vi "Evaluate Concentration.vi"(5 "python in":refnum<k35>, 6 "List Concentration In":T1(array[cluster]) {"N. Peak" items=["0.000000", "1.000000", "2.000000", "3.000000", "4.000000", "5.000000", "6.000000", "7.000000", "8.000000", "9.000000", "10.000000", "11.000000", "12.000000", "13.000000", "14.000000", "15.000000", "16.000000", "17.000000", "18.000000", "19.000000", "20.000000", "21.000000", "22.000000", "23.000000", "24.000000", "25.000000", "26.000000", "27.000000", "28.000000"]}, 7 "Type Conentration":enum32{"Item 0", "Item 1"}(radio), 8 "error in":errorcluster, 9 "List ROI in":dbl[][](array[numeric]), 10 "Parameters In":T3[](array[typedef]), 11 "Elements Selected":string[][](table)) -> (0 "error out":errorcluster, 3 "Concentration":T2, 4 "python out":refnum<k35>)   [LabVIEW 2023]
uses:
  control/Parameters.ctl
  control/Concentrations.ctl
  e2a7fa98-077b-4280-a056-373c7a60fd3a.vi
  1848effe-5ca7-4314-be89-901603a86480.vi
  8bf43f8d-2068-40c8-874a-5f9a9f6e8e88.vi
  <vilib>/Comparison/Equal/Equal Functor/Equal Functor.lvclass
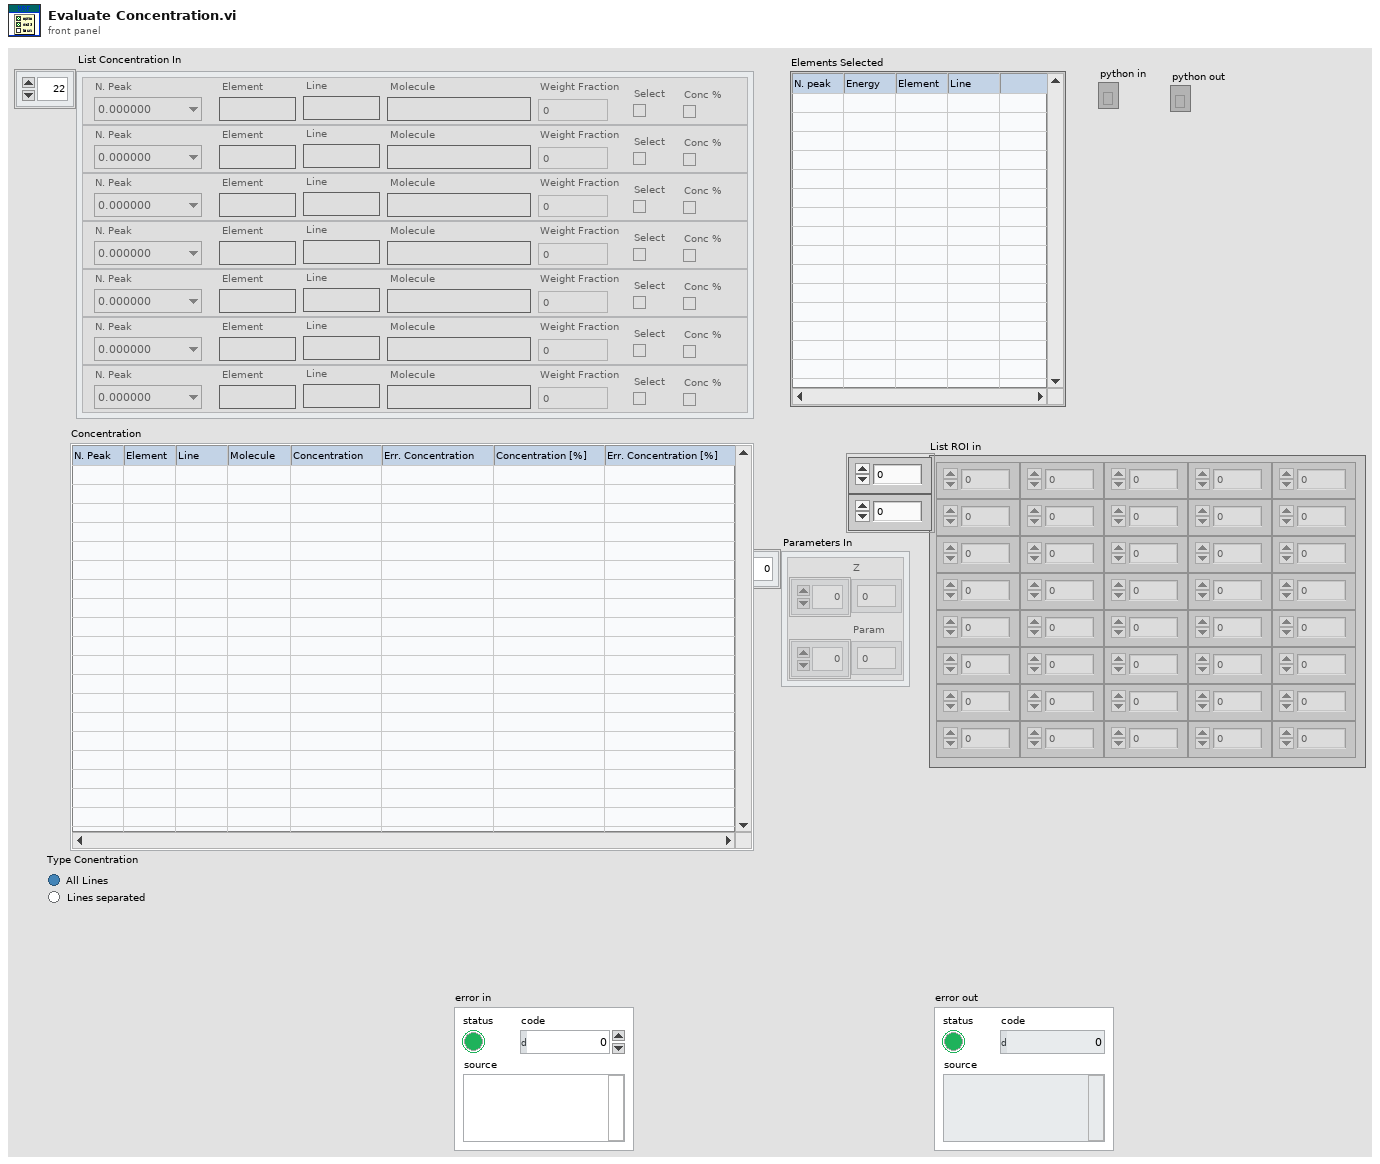
[diagram p1: front panel]
types:
  T1 = cluster{"N. Peak":u16, "Element":string, "Molecule":string, "Weight Fraction":dbl, "Select":bool, "Conc %":bool, "Line":string}[]
  T2 = typedef "Concentrations.ctl" = string[][]
  T3 = typedef "Parameters.ctl" = cluster{"Z":i32[], "Param":dbl[]}
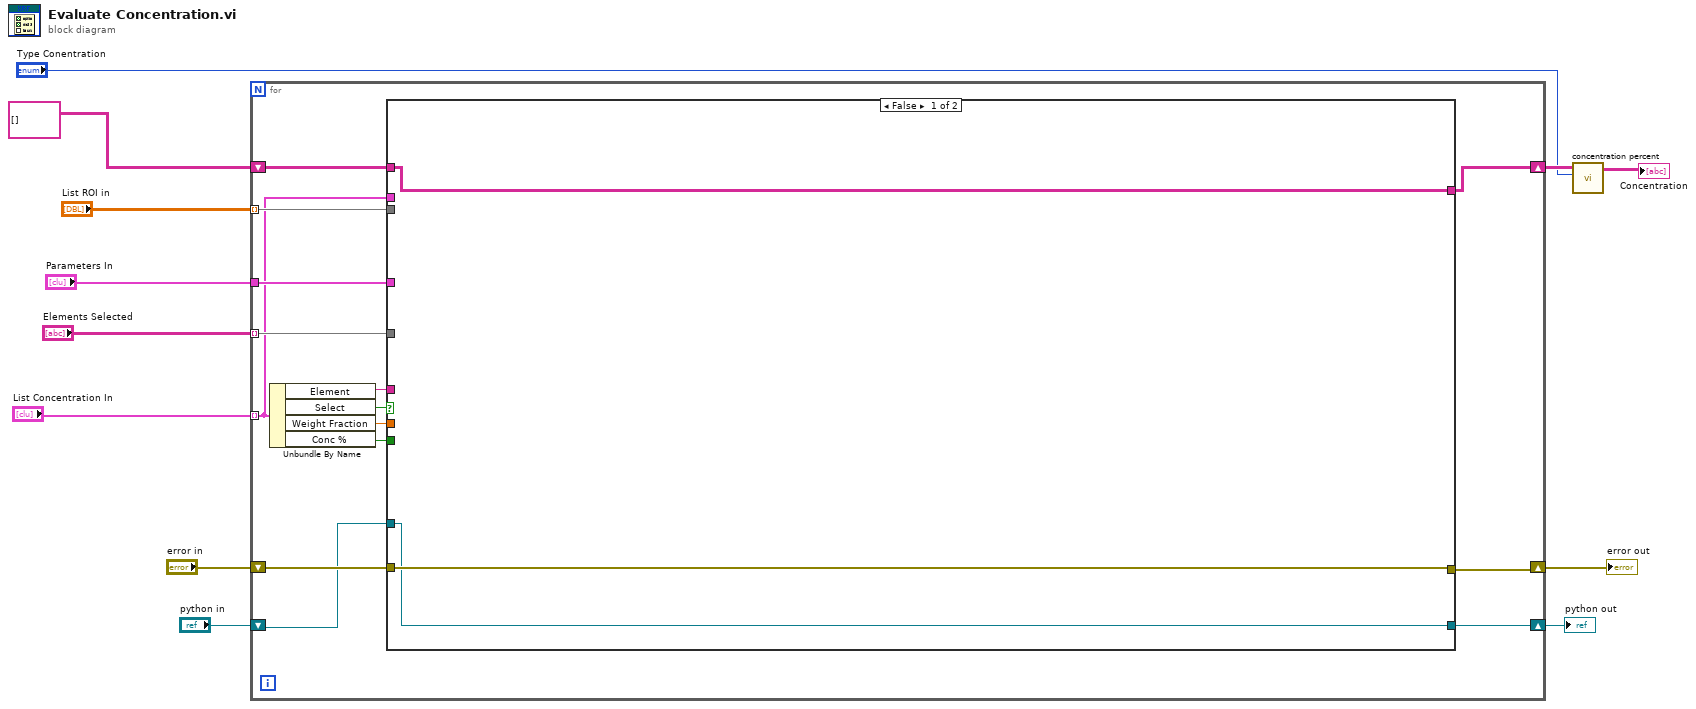
[diagram p0: block diagram]
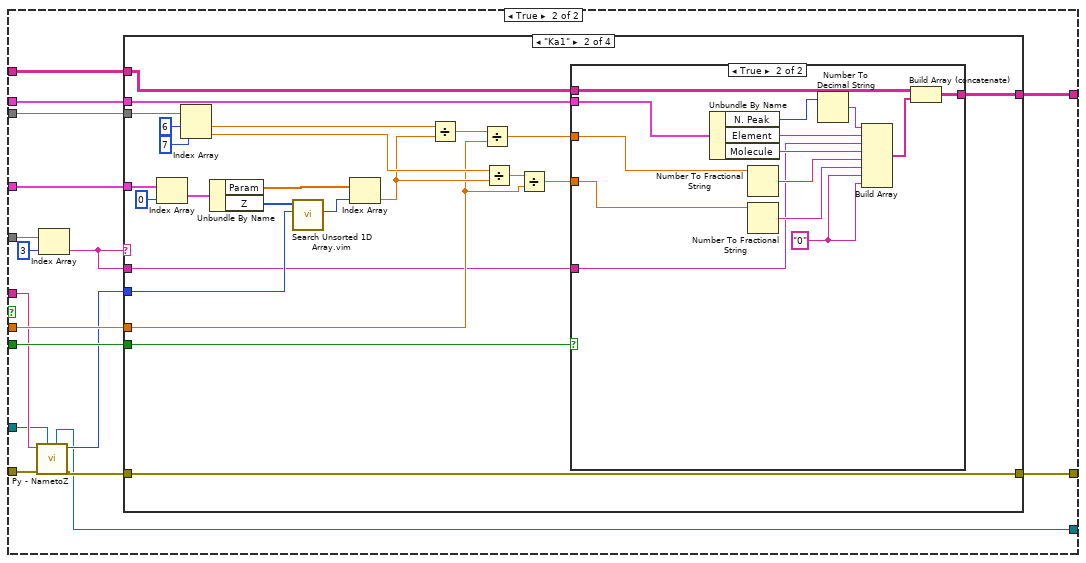
[diagram p2: hidden frame]
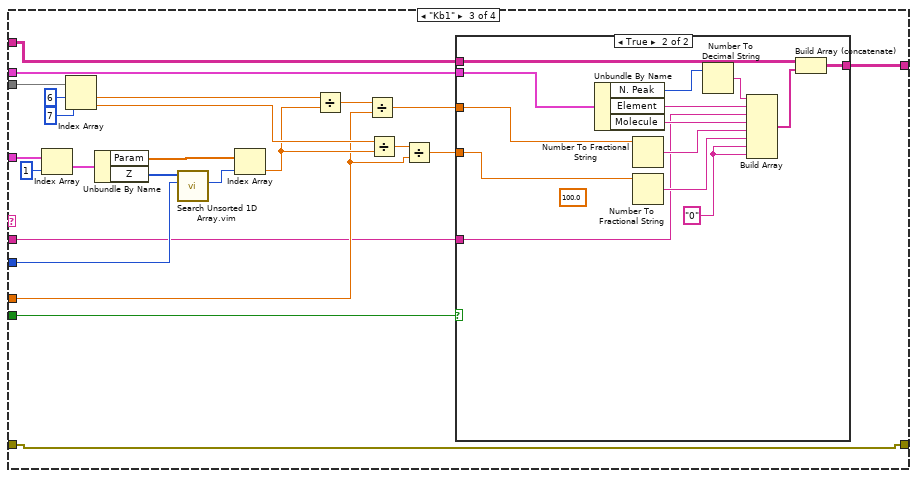
[diagram p5: hidden frame]
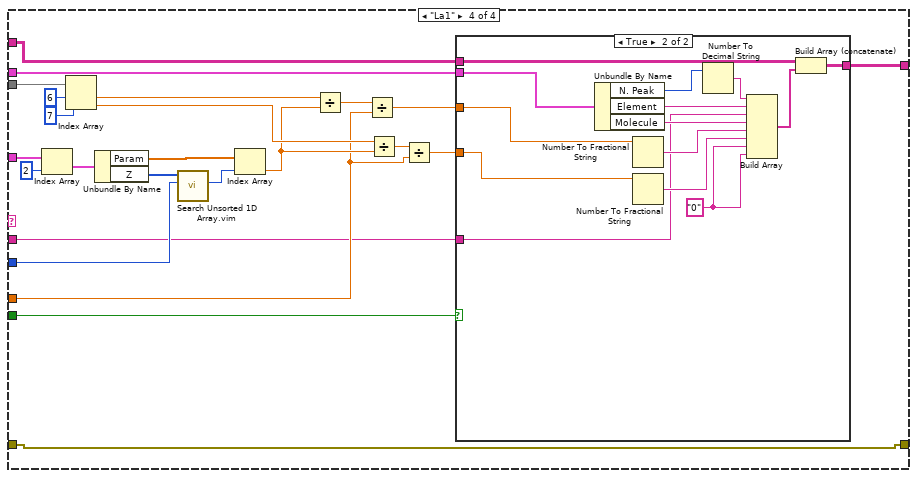
[diagram p7: hidden frame]
diagram:
  n1 = for {
    tunnel: "List Concentration In" -> [w18] mode=indexing
    tunnel: "Elements Selected" -> [w25] mode=indexing
    tunnel: "Parameters In" -> [w24]
    tunnel: "List ROI in" -> [w22] mode=indexing
    shift-right: [w17] -> w8
    shift-left: T2 [] ("Concentration") -> [w19]
    shift-right: [w15] -> w3
    shift-left: "error in" -> [w16]
    shift-right: [w14] -> w2
    shift-left: "python in" -> [w13]
    n2 = Unbundle By Name(w18) -> ("Element"=w23:string, "Select"=w26:bool, "Weight Fraction"=w21:dbl, "Conc %"=w20:bool)
    n3 = case shown="False" w26 {
      tunnel: w25 -> [_ w46]
      tunnel: w24 -> [_ w44]
      tunnel: w23 -> [_ w33]
      tunnel: w22 -> [_ w43]
      tunnel: w21 -> [_ w42]
      tunnel: w20 -> [_ w41]
      tunnel: w19 -> [w29 w40]
      tunnel: w18 -> [_ w39]
      tunnel: [w29 w38] -> w17
      tunnel: w16 -> [w28 w35]
      tunnel: [w28 w36] -> w15
      tunnel: [w27 w31] -> w14
      tunnel: w13 -> [w27 w30]
      frame False {
      }
      frame True {
        n4 = call "Py - NametoZ.vi"("python in"=w30, "error in"=w35, "Name Element"=w33) -> ("error out"=w34:errorcluster, "Z"=w32:i32, "python out"=w31:refnum<k35>)  [unwired: 6 in]
        n5 = Index Array(array=w46, index=3) -> (element=w37:string)
        n6 = case shown="\"Ka1\"" w37 {
          tunnel: w44 -> [_ w72 w111 w150]
          tunnel: w32 -> [_ w69 w108 w147]
          tunnel: w43 -> [_ w65 w104 w143]
          tunnel: w42 -> [_ w57 w96 w135]
          tunnel: w41 -> [_ w56 w95 w134]
          tunnel: w40 -> [w48 w54 w93 w132]
          tunnel: w39 -> [_ w55 w94 w133]
          tunnel: [w48 w51 w90 w129] -> w38
          tunnel: w37 -> [_ w50 w89 w128]
          tunnel: [w47 w49 w88 w127] -> w36
          tunnel: w34 -> [w47 w49 w88 w127]
          frame Default {
          }
          frame "Ka1" {
            n7 = Index Array(array=w72, index=0) -> (element=w70:T3)
            n8 = Index Array(array=w65, index #1=6 ("index"), index #2=7 ("index")) -> (element #1=w62:dbl, element #2=w59:dbl)
            n9 = Unbundle By Name(w70) -> ("Param"=w67:dbl[], "Z"=w68:i32[])
            n10 = call "Search Unsorted 1D Array.vim"("element"=w69, "unsorted 1D array"=w68) -> ("index of element"=w66:i32)  [unwired: 9 in]
            n11 = Index Array(array=w67, index=w66) -> (element=w58:dbl)
            n12 = Divide(x=w62, y=w58) -> (x/y=w61:dbl)
            n13 = Divide(x=w61, y=w57) -> (x/y=w53:dbl)
            n14 = Divide(x=w59, y=w58) -> (x/y=w60:dbl)
            n15 = Divide(x=w60, y=w57) -> (x/y=w52:dbl)
            n16 = case shown="True" w56 {
              tunnel: w55 -> [_ w87]
              tunnel: w54 -> [w73 w83]
              tunnel: [w73 w82] -> w51
              tunnel: w53 -> [_ w77]
              tunnel: w52 -> [_ w78]
              tunnel: w50 -> [_ w74]
              frame False {
              }
              frame True {
                w76 = "0"
                n17 = Unbundle By Name(w87) -> ("N. Peak"=w86:u16, "Element"=w84:string, "Molecule"=w75:string)
                n18 = Number To Fractional String(number=w77) -> (F-format string=w81:string)  [unwired: 3 in]
                n19 = Number To Fractional String(number=w78) -> (F-format string=w80:string)  [unwired: 3 in]
                n20 = Number To Decimal String(number=w86) -> (decimal integer string=w85:string)  [unwired: 1 in]
                n21 = Build Array(w85, w84, w74, w75, w81, w80, w76, w76) -> (w79:string[])
                n22 = Build Array (concatenate)(w83, w79) -> (w82:T2)
              }
            }
          }
          frame "Kb1" {
            n23 = Index Array(array=w111, index=1) -> (element=w109:T3)
            n24 = Index Array(array=w104, index #1=6 ("index"), index #2=7 ("index")) -> (element #1=w101:dbl, element #2=w98:dbl)
            n25 = Unbundle By Name(w109) -> ("Param"=w106:dbl[], "Z"=w107:i32[])
            n26 = call "Search Unsorted 1D Array.vim"("element"=w108, "unsorted 1D array"=w107) -> ("index of element"=w105:i32)  [unwired: 9 in]
            n27 = Index Array(array=w106, index=w105) -> (element=w97:dbl)
            n28 = Divide(x=w101, y=w97) -> (x/y=w100:dbl)
            n29 = Divide(x=w100, y=w96) -> (x/y=w92:dbl)
            n30 = Divide(x=w98, y=w97) -> (x/y=w99:dbl)
            n31 = Divide(x=w99, y=w96) -> (x/y=w91:dbl)
            n32 = case shown="True" w95 {
              tunnel: w94 -> [_ w126]
              tunnel: w93 -> [w112 w121]
              tunnel: [w112 w120] -> w90
              tunnel: w92 -> [_ w115]
              tunnel: w91 -> [_ w116]
              tunnel: w89 -> [_ w113]
              frame False {
              }
              frame True {
                w114 = "0" ("element")
                (unwired) 100.0 ("x")
                n33 = Unbundle By Name(w126) -> ("N. Peak"=w125:u16, "Element"=w123:string, "Molecule"=w122:string)
                n34 = Number To Fractional String(number=w115) -> (F-format string=w119:string)  [unwired: 3 in]
                n35 = Number To Fractional String(number=w116) -> (F-format string=w118:string)  [unwired: 3 in]
                n36 = Number To Decimal String(number=w125) -> (decimal integer string=w124:string)  [unwired: 1 in]
                n37 = Build Array(w124, w123, w113, w122, w119, w118, w114, w114) -> (w117:string[])
                n38 = Build Array (concatenate)(w121, w117) -> (w120:T2)
              }
            }
          }
          frame "La1" {
            n39 = Index Array(array=w150, index=2) -> (element=w148:T3)
            n40 = Index Array(array=w143, index #1=6 ("index"), index #2=7 ("index")) -> (element #1=w140:dbl, element #2=w137:dbl)
            n41 = Unbundle By Name(w148) -> ("Param"=w145:dbl[], "Z"=w146:i32[])
            n42 = call "Search Unsorted 1D Array.vim"("element"=w147, "unsorted 1D array"=w146) -> ("index of element"=w144:i32)  [unwired: 9 in]
            n43 = Index Array(array=w145, index=w144) -> (element=w136:dbl)
            n44 = Divide(x=w140, y=w136) -> (x/y=w139:dbl)
            n45 = Divide(x=w139, y=w135) -> (x/y=w131:dbl)
            n46 = Divide(x=w137, y=w136) -> (x/y=w138:dbl)
            n47 = Divide(x=w138, y=w135) -> (x/y=w130:dbl)
            n48 = case shown="True" w134 {
              tunnel: w133 -> [_ w165]
              tunnel: w132 -> [w151 w160]
              tunnel: [w151 w159] -> w129
              tunnel: w131 -> [_ w154]
              tunnel: w130 -> [_ w155]
              tunnel: w128 -> [_ w152]
              frame False {
              }
              frame True {
                w153 = "0" ("F-format string")
                n49 = Unbundle By Name(w165) -> ("N. Peak"=w164:u16, "Element"=w162:string, "Molecule"=w161:string)
                n50 = Number To Fractional String(number=w154) -> (F-format string=w158:string)  [unwired: 3 in]
                n51 = Number To Fractional String(number=w155) -> (F-format string=w157:string)  [unwired: 3 in]
                n52 = Number To Decimal String(number=w164) -> (decimal integer string=w163:string)  [unwired: 1 in]
                n53 = Build Array(w163, w162, w152, w161, w158, w157, w153, w153) -> (w156:string[])
                n54 = Build Array (concatenate)(w160, w156) -> (w159:T2)
              }
            }
          }
        }
      }
    }
  }
  "error out" <- w3
  "python out" <- w2
  n55 = call "concentration percent.vi"("Type Conentration"="Type Conentration", "Concentration In"=w8) -> ("Concentration Out"=→"Concentration":T2)  [unwired: 9 in]
